vi "setFlyBehavior.vi"(8 "error in (no error)":errorcluster, 10 "FlyBehavior.lvclass":refnum<class "FlyBehavior.lvclass">, 11 "Duck in":refnum<class "Duck.lvclass">) -> (0 "error out":errorcluster, 3 "Duck out":refnum<class "Duck.lvclass">)   [LabVIEW 2013, in "Duck.lvclass"]
uses:
  Duck.lvclass
  FlyBehavior/FlyBehavior.lvclass
  Duck.lvclass/Duck.ctl
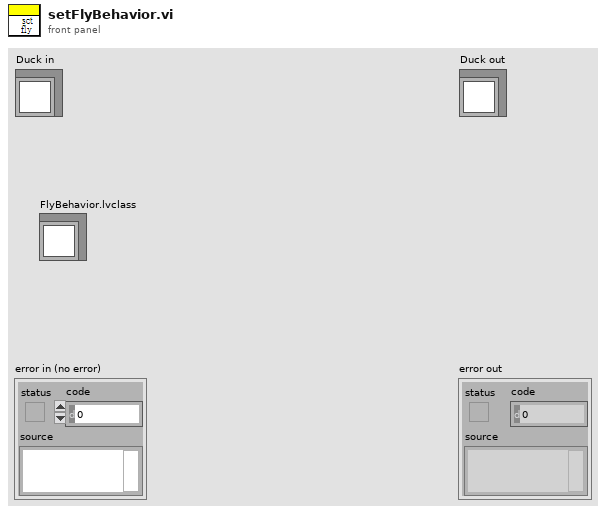
[diagram p1: front panel]
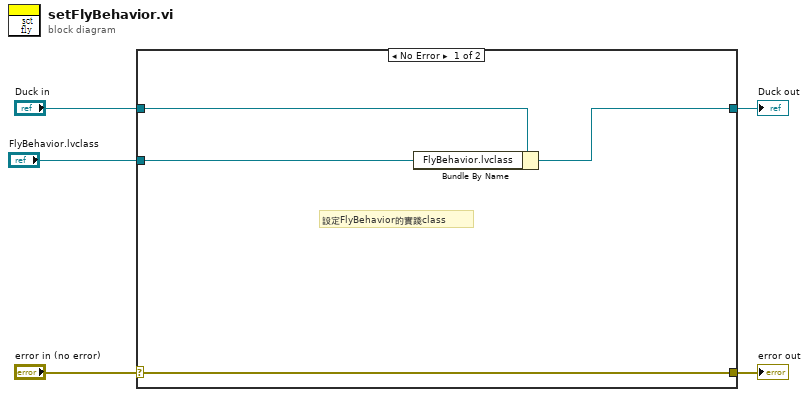
[diagram p0: block diagram]
diagram:
  n1 = case shown="No Error" "error in (no error)" {
    selector: "error in (no error)" -> [w9 w11]
    tunnel: [w9 w11] -> w4
    tunnel: [w6 w10] -> w2
    tunnel: "Duck in" -> [w7 w10]
    tunnel: "FlyBehavior.lvclass" -> [w8 _]
    frame No Error {
      # "設定FlyBehavior的實踐class"
      n2 = Bundle By Name(cluster=w7, "FlyBehavior.lvclass"=w8) -> (w6:refnum<class "Duck.lvclass">)
    }
    frame Error {
    }
  }
  "error out" <- w4
  "Duck out" <- w2
